vi "Bounds.vi"(1 "XRef":refnum<vi>, 2 "State In":T2) -> (0 "Bounds":cluster{"Width":T1, "Height":T1})   [LabVIEW 2018, in "Array Dimension Array.xnode"]
uses:
  Array Dimension Array.xnode
  State.ctl
  <vilib>/XNodeSupport/XNodeInt.ctl
  <vilib>/XNodeSupport/NI_XNodeSupport.lvlib
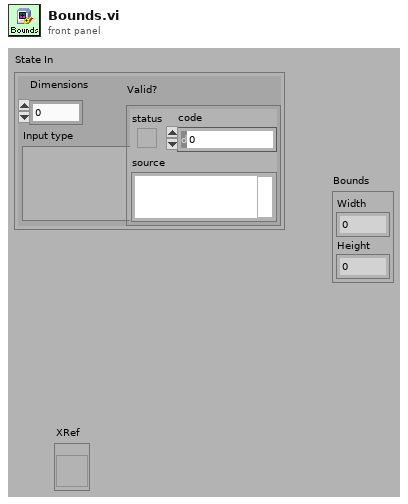
[diagram p1: front panel]
types:
  T1 = typedef "NI_XNodeSupport.lvlib/XNodeInt.ctl" = i32
  T2 = typedef "Array Dimension Array.xnode/State.ctl" = cluster{"Input type":variant, "Valid?":errorcluster, "Dimensions":i32}
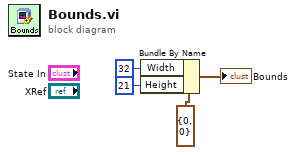
[diagram p0: block diagram]
diagram:
  n1 = Bundle By Name(cluster=cluster{"Width":T1, "Height":T1} {"Width"=0, "Height"=0} ("Bounds"), "Width"=T1 32, "Height"=T1 21) -> (→"Bounds":cluster{"Width":T1, "Height":T1})
